vi "set_timeout.vi"(11 "iteration count":i32) -> (3 "timout value":i32)   [LabVIEW 2024]
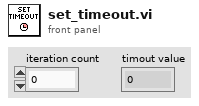
[diagram p1: front panel]
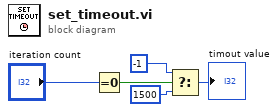
[diagram p0: block diagram]
diagram:
  n1 = Equal To 0?(x="iteration count") -> (x = 0?=w3:bool)
  n2 = Select(t=-1 ("byte count"), s=w3, f=1500) -> (s? t:f=→"timout value":i32)
